vi "Set_Notification.vi"(0 "Serial In":refnum<visa-resource-name>, 5 "Node":u8, 7 "Mode":enum16{"Position", "Velocity"}(ring), 9 "Value":i64, 11 "Error In":errorcluster) -> (4 "Serial Out":refnum<visa-resource-name>, 15 "Error Out":errorcluster)   [LabVIEW 2019]
uses:
  <vilib>/Instr/_visa.llb/Select Event Type.ctl
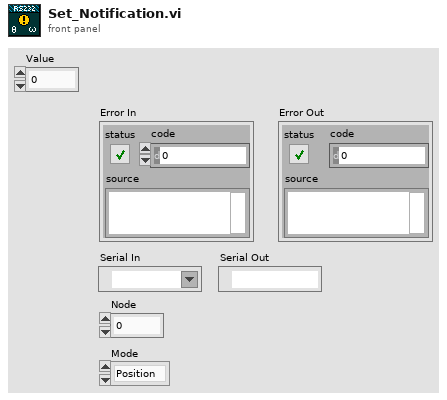
[diagram p1: front panel]
types:
  T1 = typedef "Select Event Type.ctl" = u32
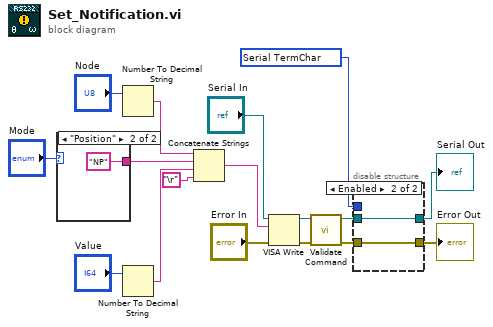
[diagram p0: block diagram]
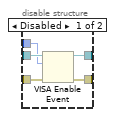
[diagram p2: hidden frame]
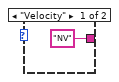
[diagram p3: hidden frame]
diagram:
  w1 = T1 1073684516 items=["Service Request"=1073684491, "Trigger"=3221168138, "Clear"=1073684493, "VXI Signal"=1073684512, "VXI/VME Interrupt"=3221168161, "VXI/VME Sysfail"=1073684509, "VXI/VME Sysreset"=1073684510, "GPIB CIC"=1073684498, "GPIB Talk"=1073684499, "GPIB Listen"=1073684500, "PXI Interrupt"=1073684514, "Serial Break"=1073684515, "Serial TermChar"=1073684516, "Serial CTS"=1073684521, "Serial DSR"=1073684522, "Serial DCD"=1073684524, "Serial RI"=1073684526, "Serial Character"=1073684533, "USB Interrupt"=1073684535, "All Enabled"=1073709055] ("Event Type")
  n1 = case shown="\"Position\"" "Mode" {
    tunnel: ["NV" ("string") "NP" ("string")] -> w12
    frame "Velocity" {
    }
    frame "Position" {
    }
  }
  n2 = Number To Decimal String(number="Node") -> (decimal integer string=w14:string)  [unwired: 1 in]
  n3 = Number To Decimal String(number="Value") -> (decimal integer string=w7:string)  [unwired: 1 in]
  n4 = Concatenate Strings(w14, w12, w7, "\r") -> (w13:string)
  n5 = VISA Write(VISA resource name="Serial In", write buffer=w13, error in (no error)="Error In") -> (VISA resource name out=w11:refnum<visa-resource-name>, error out=w10:errorcluster)  [unwired: 1 out]
  n6 = call "Validate Command.vi"("error in (no error)"=w10, "Serial in"=w11) -> ("error out"=w2:errorcluster, "Serial Out"=w5:refnum<visa-resource-name>)  [unwired: 3 in, 1 out]
  n7 = disable-structure shown="Enabled" {
    disable-tunnel: w5 -> [w24 w26]
    disable-tunnel: [w23 w26] -> w4
    disable-tunnel: [w22 w25] -> w3
    disable-tunnel: w2 -> [w21 w25]
    disable-tunnel: w1 -> [w20 _]
    frame Disabled {
      n8 = VISA Enable Event(8:w21, 10:w20, 11:w24) -> (0:w22:errorcluster, 3:w23:refnum<visa-resource-name>)  [unwired: 1 in]
    }
    frame Enabled {
    }
  }
  "Error Out" <- w3
  "Serial Out" <- w4
